vi "reset.vi"(8 "error in (no error)":errorcluster) -> (0 "error out":errorcluster)   [LabVIEW 2014]
uses:
  Controls/Track Controls.ctl
  Controls/Track Volume Settings.ctl
  Sub VIs/Audio/Controls/playback state.ctl
  Controls/Application Data.vi
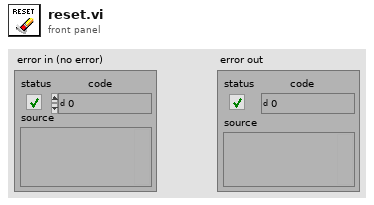
[diagram p1: front panel]
types:
  T1 = typedef "playback state.ctl" = enum16{"Load File", "Save File", "Play", "Record", "Stop", "Rewind"}
  T2 = typedef "Track Controls.ctl" = cluster{"Track 0":T3, "Track 1":T3, "Track 2":T3, "Track 3":T3}
  T3 = typedef "Track Volume Settings.ctl" = cluster{"Volume":dbl, "Pan":dbl, "Record":bool, "FX":bool}
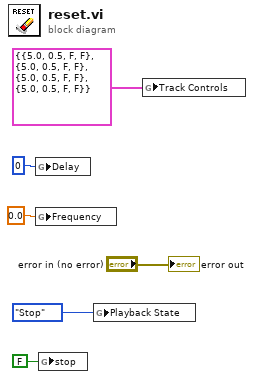
[diagram p0: block diagram]
diagram:
  n1 = global write "Application Data.vi" "Delay"(u32 0 ("Delay")) -> ()
  n2 = global write "Application Data.vi" "Frequency"(0.0 ("Frequency")) -> ()
  n3 = global write "Application Data.vi" "stop"(FALSE ("stop")) -> ()
  n4 = global write "Application Data.vi" "Playback State"(playback_state."Stop" ("Playback State")) -> ()
  n5 = global write "Application Data.vi" "Track Controls"(T2 {"Track 0"={"Volume"=5.0, "Pan"=0.5, "Record"=FALSE, "FX"=FALSE}, "Track 1"={"Volume"=5.0, "Pan"=0.5, "Record"=FALSE, "FX"=FALSE}, "Track 2"={"Volume"=5.0, "Pan"=0.5, "Record"=FALSE, "FX"=FALSE}, "Track 3"={"Volume"=5.0, "Pan"=0.5, "Record"=FALSE, "FX"=FALSE}} ("Track Controls 2")) -> ()
  "error out" <- "error in (no error)"
